vi "test_Set Instrument Addon Name.vi"(8 "error in (no error)":errorcluster, 11 "TestCase in":refnum<class "Instrument Addon Scripting API Custom Device Unit Tests.lvclass">) -> (0 "error out":errorcluster, 3 "TestCase out":refnum<class "Instrument Addon Scripting API Custom Device Unit Tests.lvclass">)   [LabVIEW 2018, in "Instrument Addon Scripting API Custom Device Unit Tests.lvclass"]
uses:
  Instrument Addon Scripting API Custom Device Unit Tests.lvclass
  <vilib>/addons/_JKI Toolkits/VI Tester/TestCase.llb/TestCase.lvclass
  Instrument Addon Scripting API Test Assets/Instrument Addon Scripting API Test Assets.lvclass
  APIs/Scripting API/Instrument Addon Scripting API.lvlib
  C:/Program Files (x86)/National Instruments/LabVIEW 2018/vi.lib/addons/_JKI Toolkits/VI Tester/TestCase.llb/TestCase.lvclass
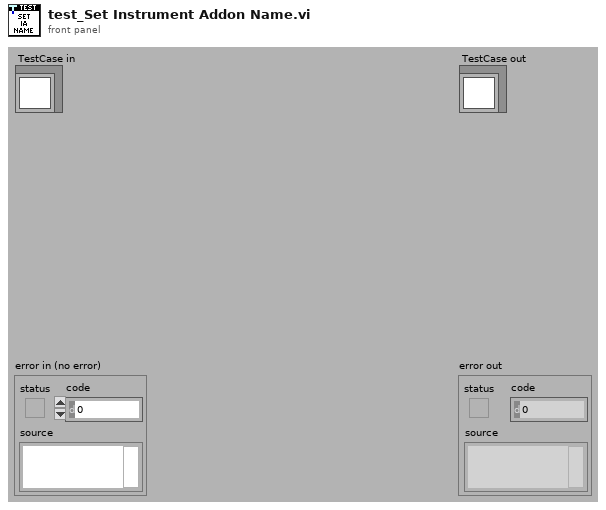
[diagram p1: front panel]
types:
  T1 = typedef "Custom Device API.lvlib/Custom Device Item Ref.ctl" = u64
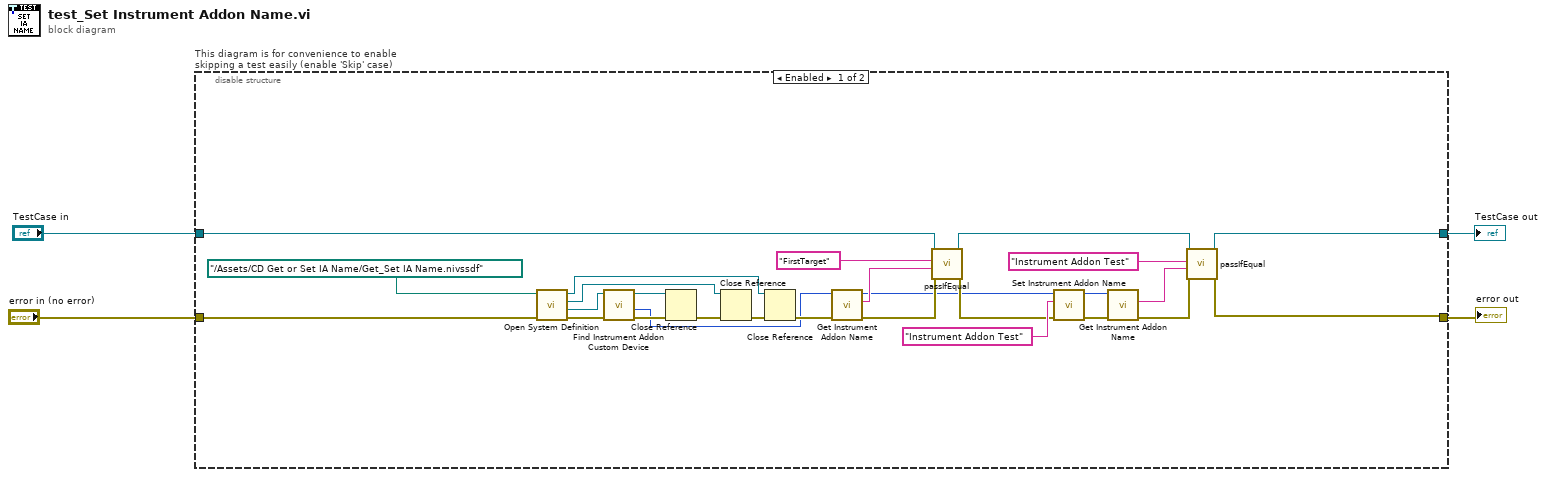
[diagram p0: block diagram]
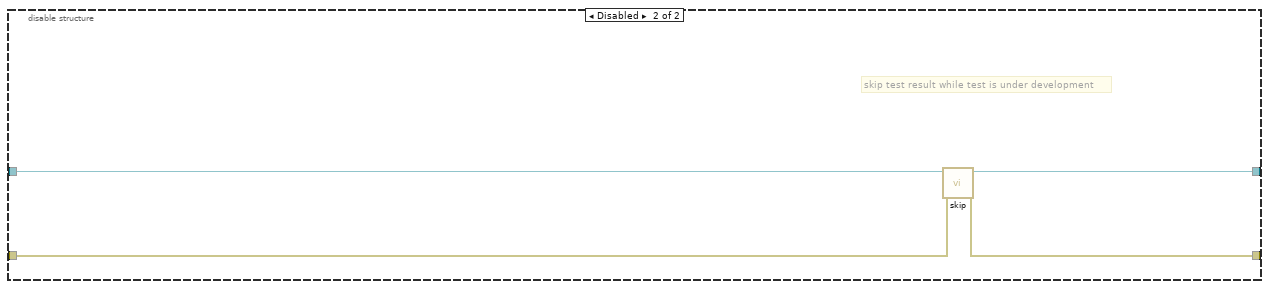
[diagram p2: hidden frame]
diagram:
  n1 = disable-structure "This diagram is for convenience to enable skipping a test easily (enable 'Skip' case)" shown="Enabled" {
    disable-tunnel: "TestCase in" -> [w6 w35]
    disable-tunnel: [w31 w33] -> w1
    disable-tunnel: [w30 w34] -> w3
    disable-tunnel: "error in (no error)" -> [w29 w32]
    frame Enabled {
      n2 = call "Open System Definition.vi"("error in (no error)"=w29, "System Definition File"=path "../Assets/CD Get or Set IA Name/Get_Set IA Name.nivssdf") -> ("error out"=w28:errorcluster, "Target Refnum"=w27:refnum<k24>, "Root Refnum"=w22:refnum<k24>, "System Definition Refnum"=w23:refnum<k24>)  [unwired: 6 in]
      n3 = call "Find Instrument Addon Custom Device.vi"("error in"=w28, "target in"=w27) -> ("error out"=w19:errorcluster, "NodeID"=w12:u64, "target out"=w20:refnum<k24>)  [unwired: 7 in]
      n4 = Close Reference(reference=w20, error in (no error)=w19) -> (error out=w21:errorcluster)
      n5 = Close Reference(reference=w22, error in (no error)=w21) -> (error out=w24:errorcluster)
      n6 = Close Reference(reference=w23, error in (no error)=w24) -> (error out=w13:errorcluster)
      n7 = call "Get Instrument Addon Name.vi"("Error In"=w13, "Instrument Addon Refnum In"=w12) -> ("Error Out"=w11:errorcluster, "Name"=w9:string, "Instrument Addon Refnum Out"=w7:T1)  [unwired: 7 in]
      n8 = call-dynamic "passIfEqual.vi"("error in (no error)"=w11, "y"=w9, "x"="FirstTarget" ("Name"), "TestCase in"=w6) -> ("error out"=w10:errorcluster, "TestCase out"=w5:refnum<class "Instrument Addon Scripting API Custom Device Unit Tests.lvclass">)  [unwired: 6 in]
      n9 = call "Set Instrument Addon Name.vi"("Error In"=w10, "Name"="Instrument Addon Test", "Instrument Addon Refnum In"=w7) -> ("Error Out"=w18:errorcluster, "Instrument Addon Refnum Out"=w15:T1)  [unwired: 7 in]
      n10 = call "Get Instrument Addon Name.vi"("Error In"=w18, "Instrument Addon Refnum In"=w15) -> ("Error Out"=w17:errorcluster, "Name"=w14:string)  [unwired: 7 in, 1 out]
      n11 = call-dynamic "passIfEqual.vi"("error in (no error)"=w17, "y"=w14, "x"="Instrument Addon Test", "TestCase in"=w5) -> ("error out"=w30:errorcluster, "TestCase out"=w31:refnum<class "Instrument Addon Scripting API Custom Device Unit Tests.lvclass">)  [unwired: 6 in]
    }
    frame Disabled {
      # "skip test result while test is under development"
      n12 = call <vilib>:"skip.vi"("error in (no error)"=w32, "TestCase in"=w35) -> ("error out"=w34:errorcluster, "TestCase out"=w33:refnum<class "Instrument Addon Scripting API Custom Device Unit Tests.lvclass">)  [unwired: 8 in]
    }
  }
  "error out" <- w3
  "TestCase out" <- w1
